vi "打码软件.vi"() -> ()   [LabVIEW 2014]
uses:
  <vilib>/Instr/_visa.llb/VISA Configure Serial Port (Instr).vi
  <vilib>/ptbypt/NI_PtbyPt.lvlib
panel:
  in  "监控":bool
  out "选项卡控件":enum32{"主选项卡", "监控"}(tab)
  in  "输入打标码后五位\n如：S0001":string
  in  "确定":bool
  out "当前打标码":string
  in  "手动打标":bool
  in  "停止":bool
  in  "退出":bool
  in  "PLC状态":bool
  out "串口通讯":bool
  out "PLC通讯":bool
  in  "返回":bool
  out "初始化回复":string
  out "打标模式回复":string
  out "初始条码":string
  out "打标V1写入回复":string
  out "打标V3写入回复":string
  out "开始打标写入回复":string
  out "停止打标回复":string
  in  "自动打标":bool
  out "错误输出 2":errorcluster caption="错误输出"
  out "元素":u32
  out "初始化文件回复":string
  out "打标V2写入回复":string
  out "枚举":T1
  # "SIC 打 标 软 件"
  # "自定义条码"
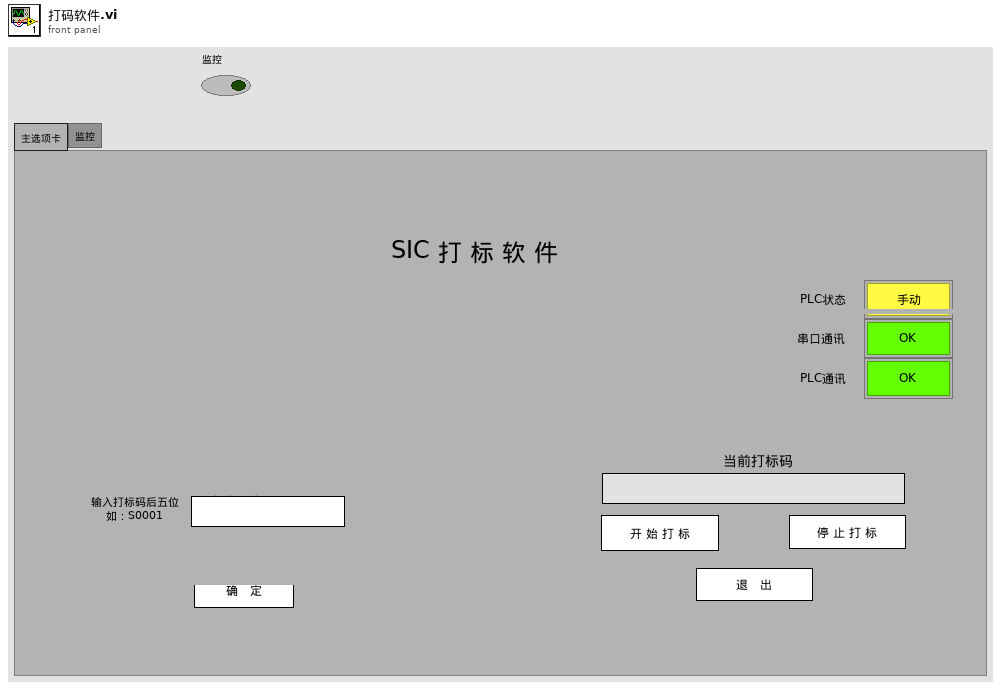
[diagram p1: front panel]
types:
  T1 = typedef "控件 1.ctl" = enum16{"通讯连接", "读PLC指令", "串口连接", "初始化", "打标模式", "事件", "错误", "退出"}
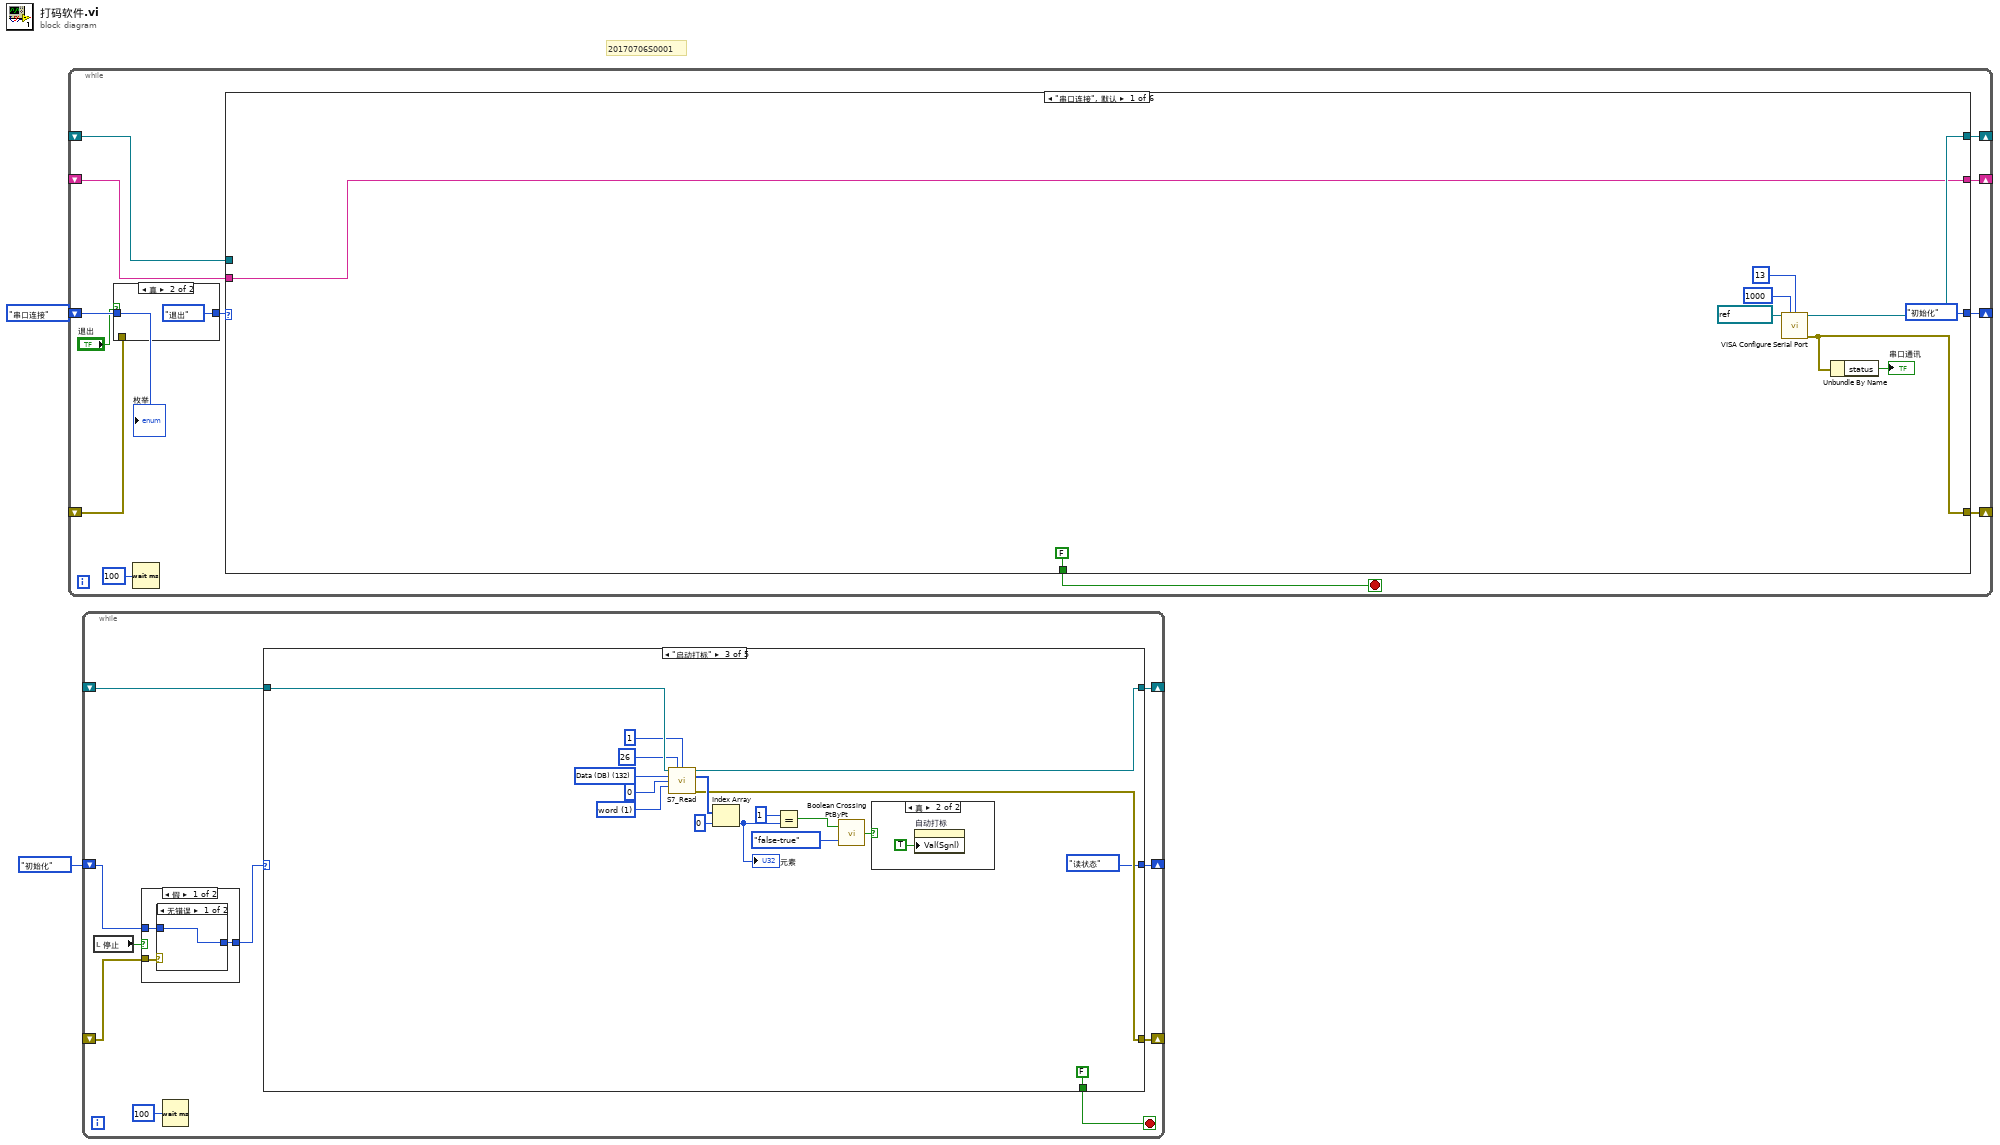
[diagram p0: block diagram]
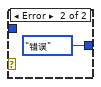
[diagram p2: hidden frame]
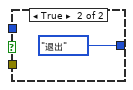
[diagram p3: hidden frame]
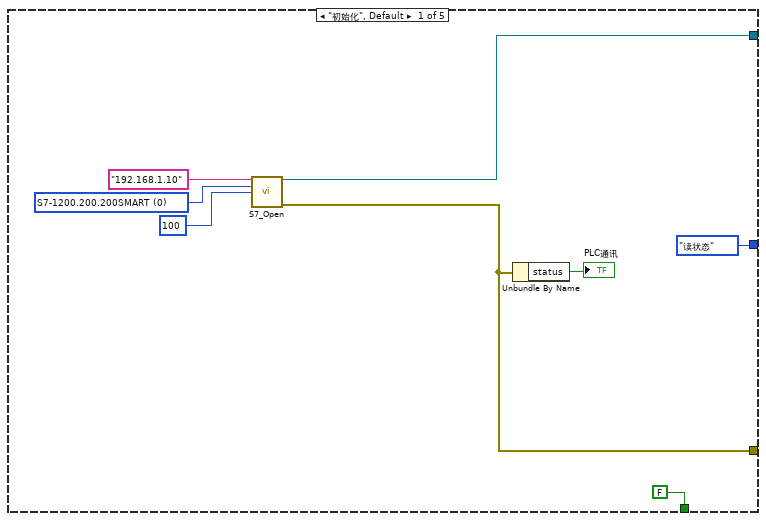
[diagram p4: hidden frame]
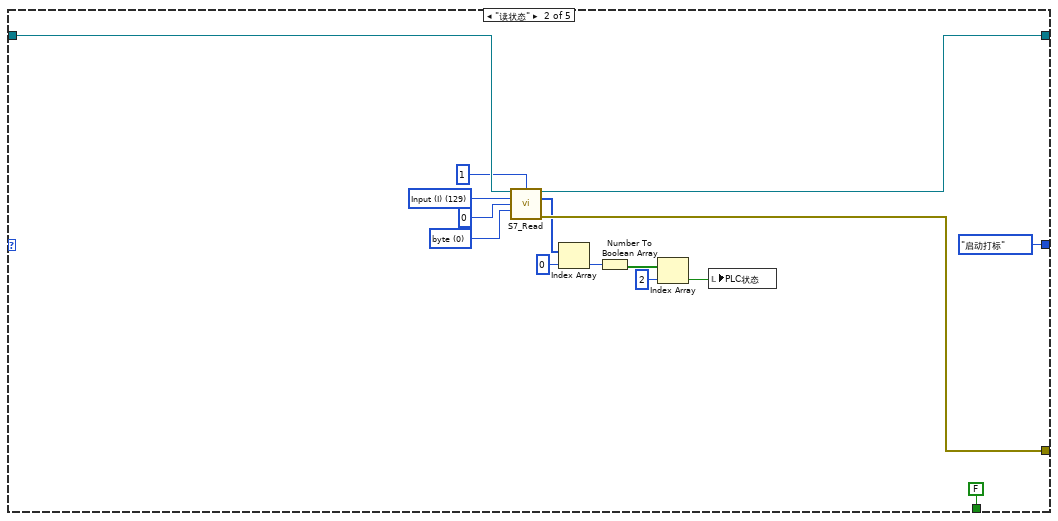
[diagram p5: hidden frame]
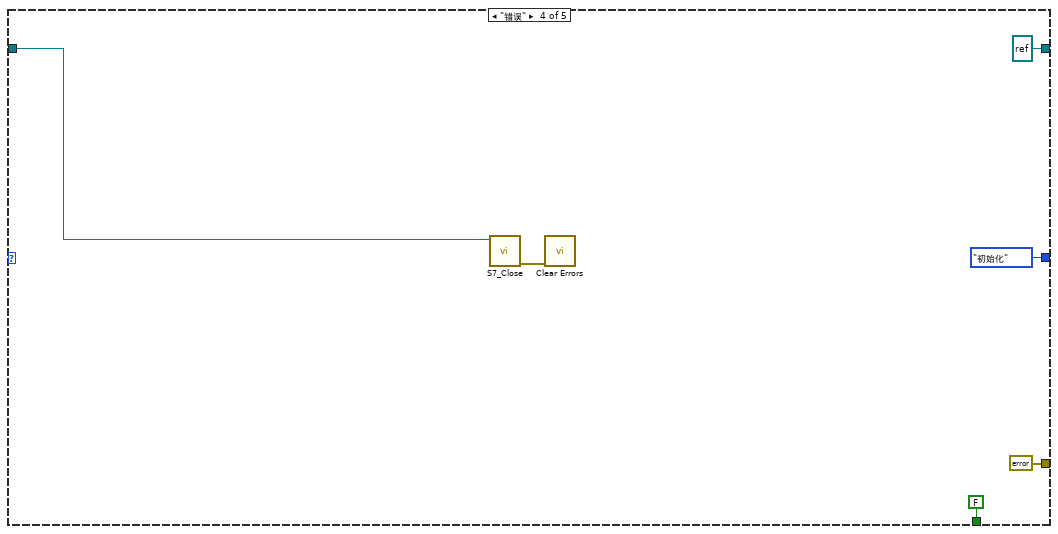
[diagram p7: hidden frame]
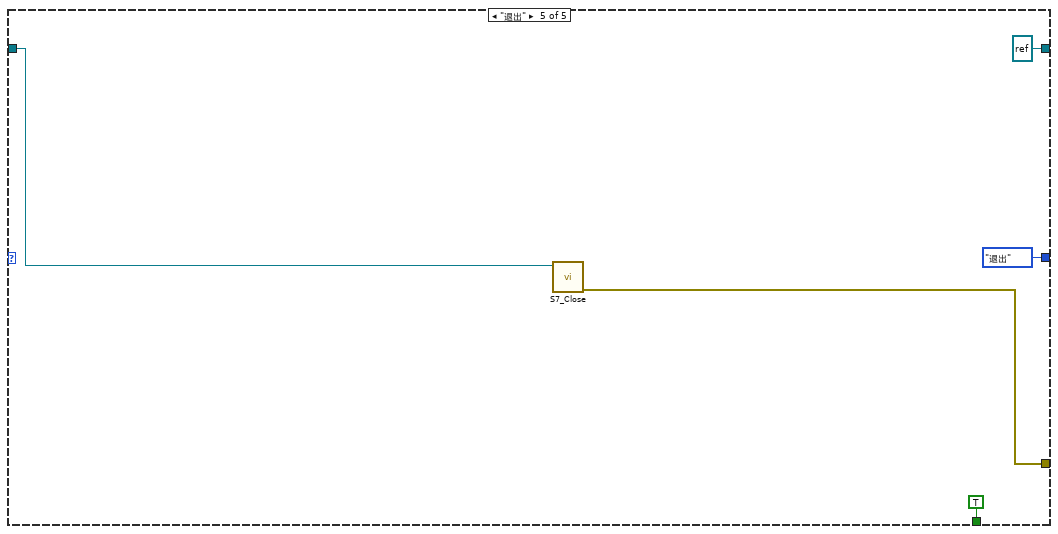
[diagram p8: hidden frame]
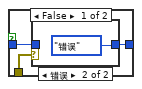
[diagram p9: hidden frame]
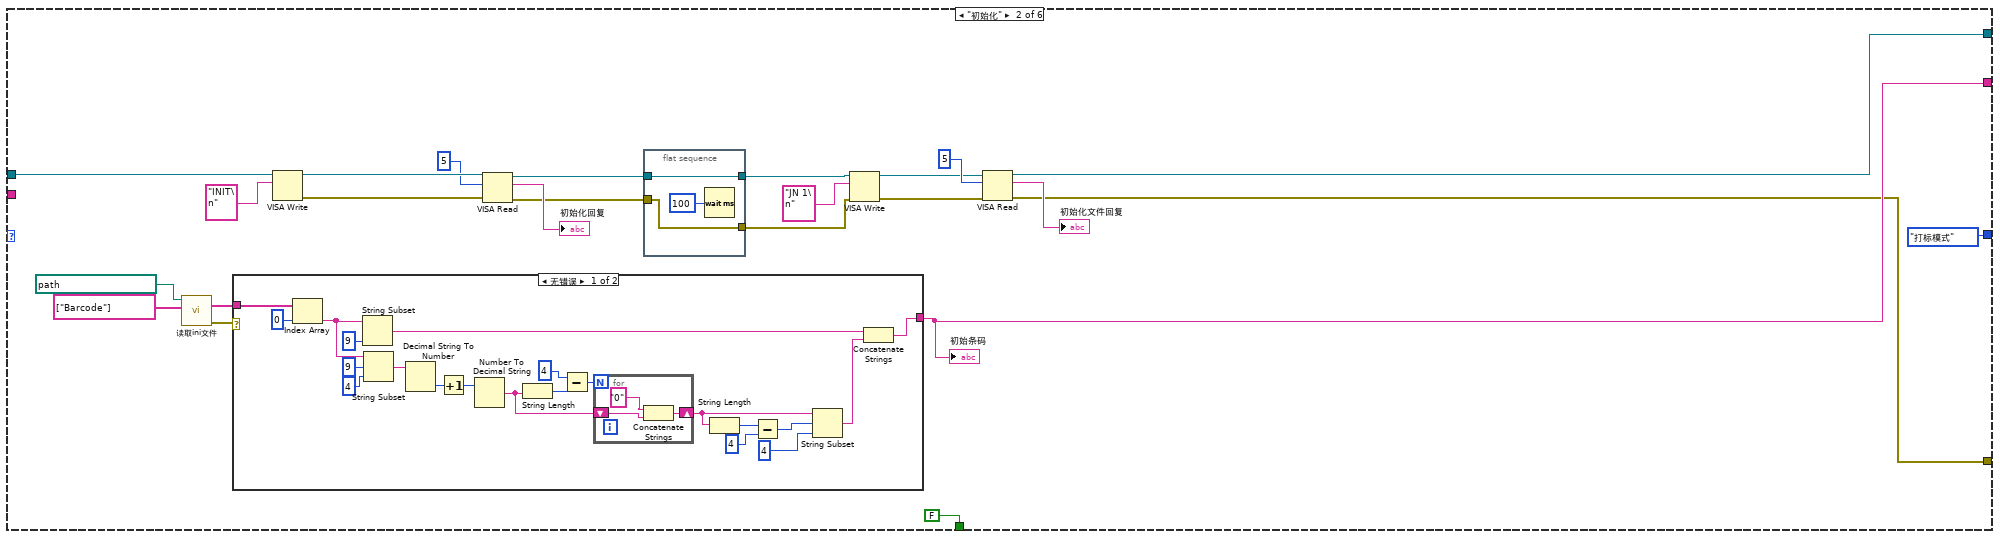
[diagram p11: hidden frame]
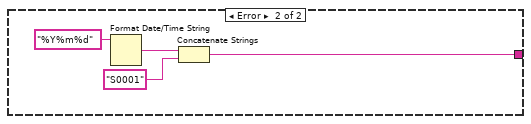
[diagram p12: hidden frame]
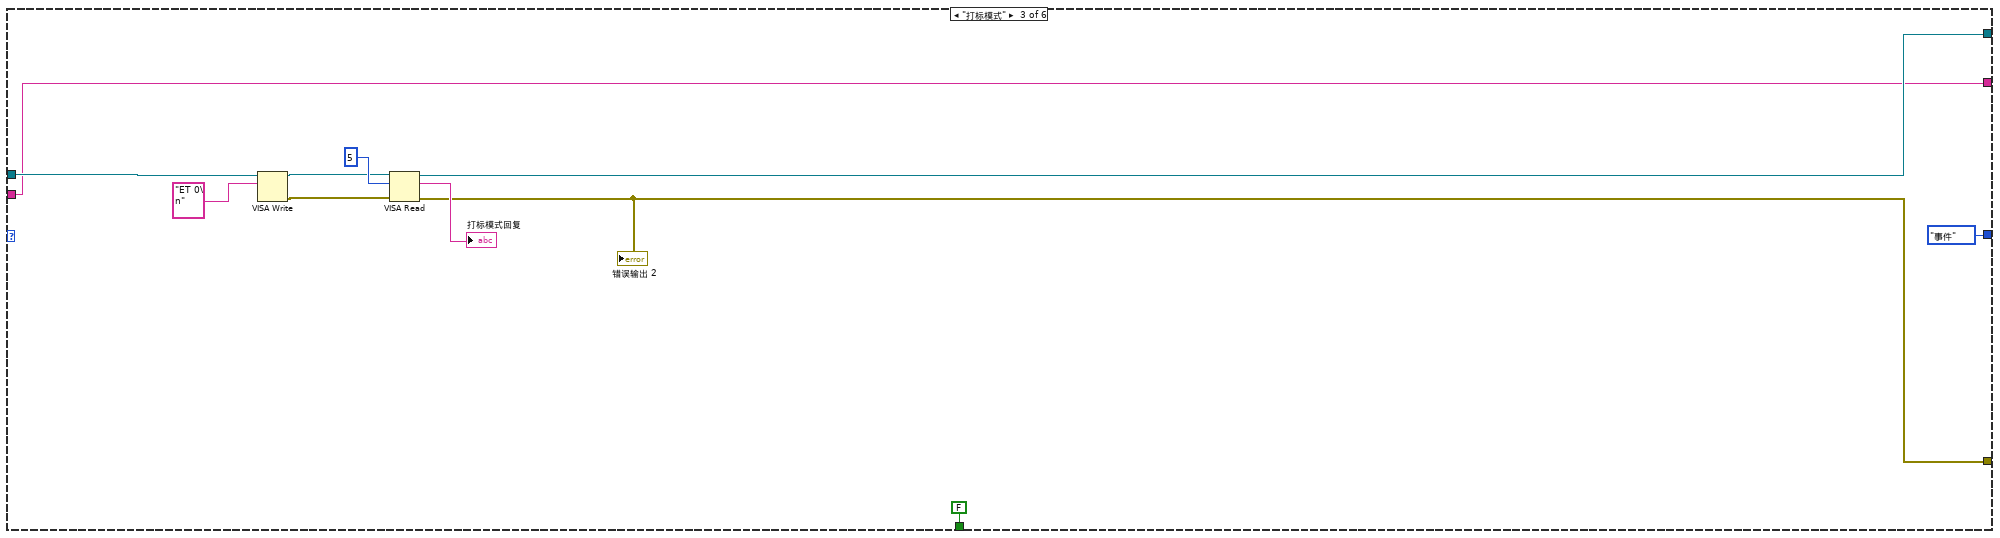
[diagram p13: hidden frame]
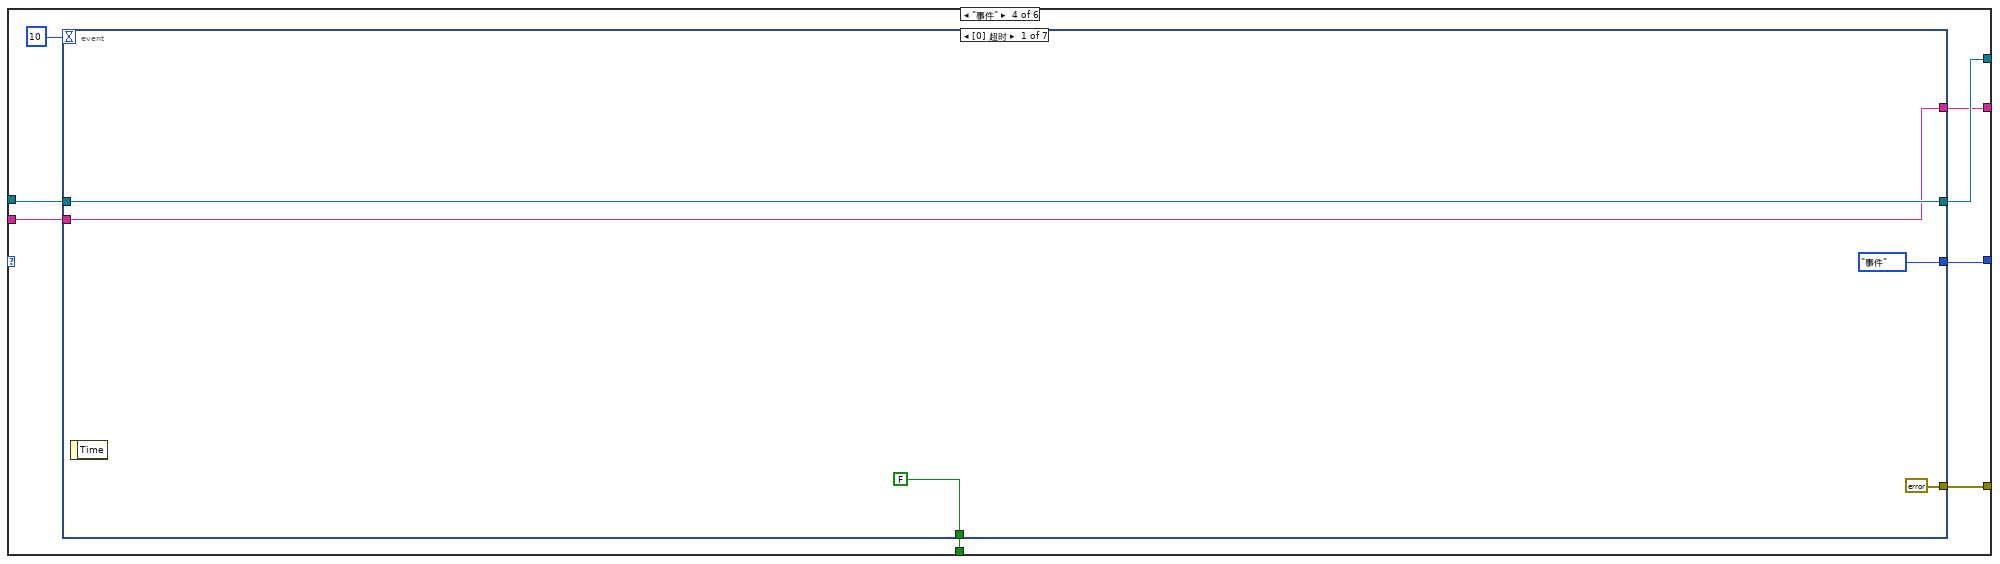
[diagram p14: hidden frame]
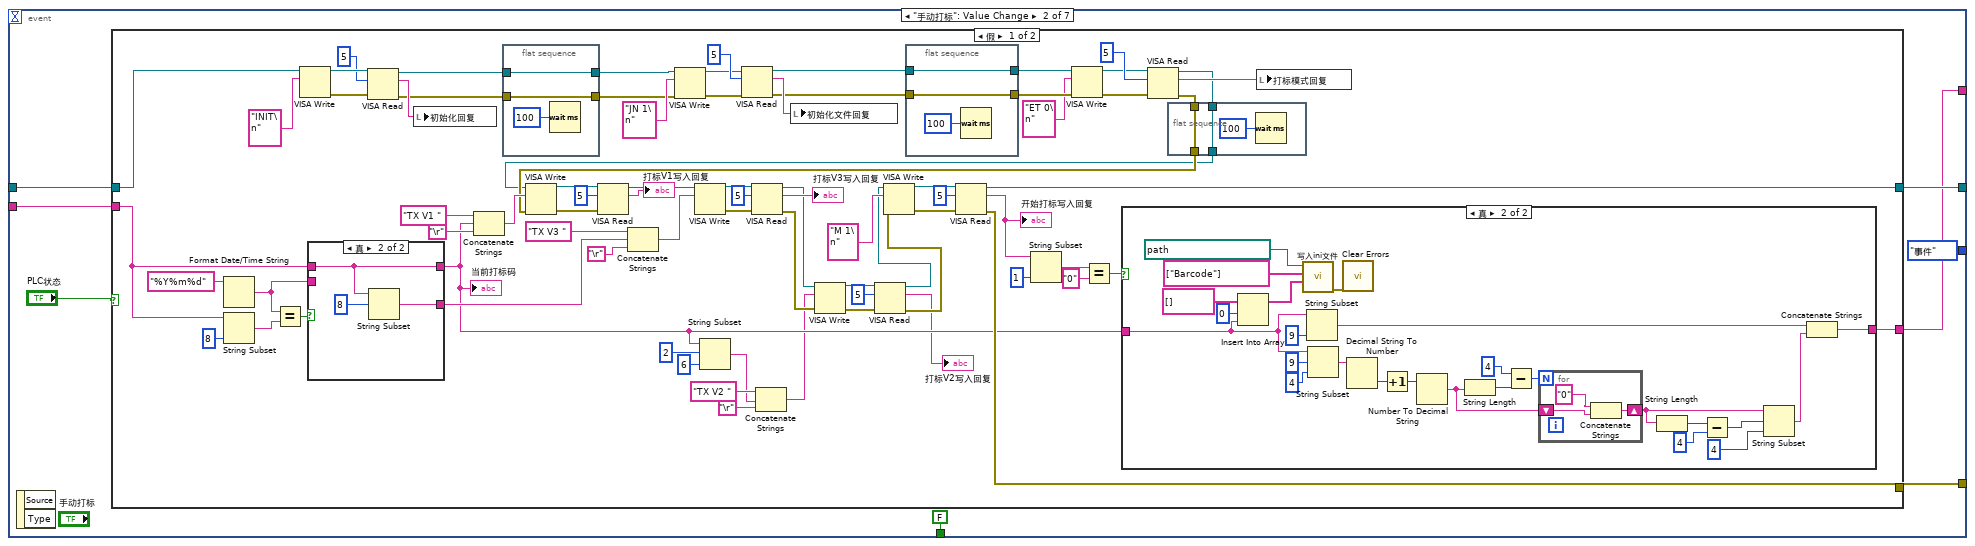
[diagram p15: hidden frame]
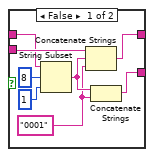
[diagram p17: hidden frame]
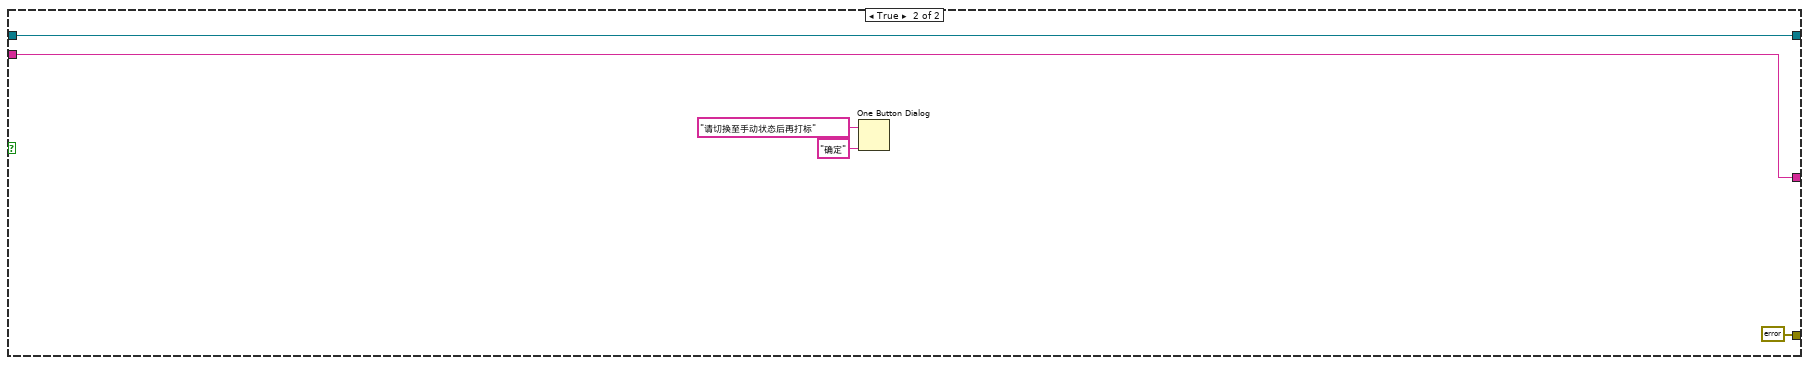
[diagram p18: hidden frame]
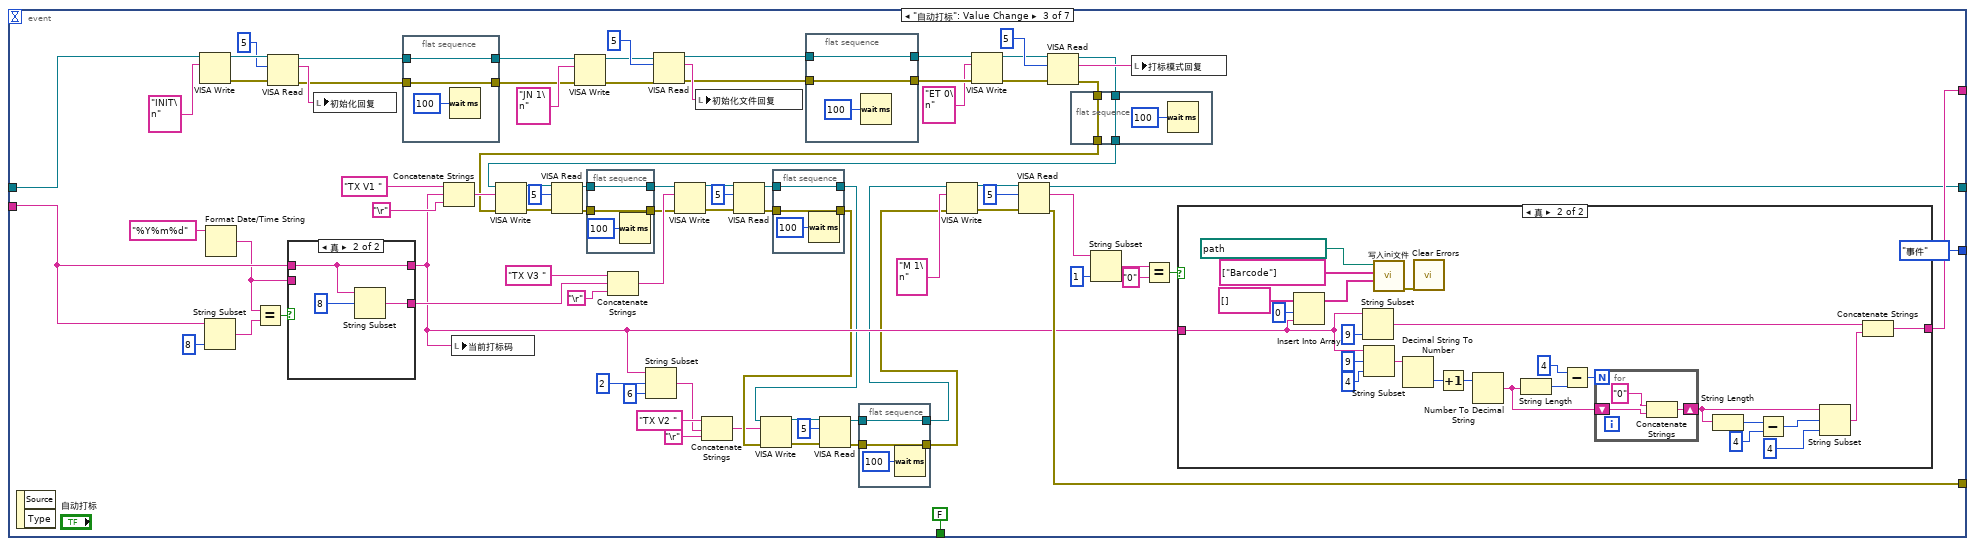
[diagram p19: hidden frame]
diagram:
  # "20170706S0001"
  n1 = while {
    shift-right: [w9] -> _
    shift-left: 控件_1."串口连接" -> [w14]
    shift-right: [w10] -> _
    shift-left: _ -> [w13]
    shift-right: [w11] -> _
    shift-left: _ -> [w8]
    shift-right: [w7] -> _
    shift-left: _ -> [w5]
    stop <- w6 stop-if-true
    n2 = case shown="真" "退出" {
      tunnel: w14 -> [w17 _]
      tunnel: w13 -> [w16 _]
      tunnel: [w15 控件_1."退出"] -> w12
      frame False {
        n3 = case shown="错误" w16 {
          tunnel: w17 -> [w18 _]
          tunnel: [w18 控件_1."错误"] -> w15
          frame No Error {
          }
          frame Error {
          }
        }
      }
      frame True {
      }
    }
    n4 = Wait (ms)(milliseconds to wait=u32 100 ("等待时间（毫秒）")) -> ()  [unwired: 1 out]
    n5 = case shown="\"串口连接\", 默认" w12 {
      tunnel: [w27 w31 w87 w99 refnum<visa-resource-name> refnum ("VISA resource name out") refnum<visa-resource-name> refnum ("VISA resource name out")] -> w11
      tunnel: [w24 w30 w88 w100 errorcluster {"status"=FALSE, "code"=0, "source"=""} ("error out") errorcluster {"status"=FALSE, "code"=0, "source"=""} ("error out")] -> w10
      tunnel: [控件_1."初始化" 控件_1."打标模式" 控件_1."事件" w97 控件_1."串口连接" 控件_1."退出"] -> w9
      tunnel: w8 -> [_ w53 w94 w102 w425 w431]
      tunnel: [w22 w42 w85 w98 w423 ""] -> w7
      tunnel: [FALSE FALSE FALSE w96 FALSE TRUE] -> w6
      tunnel: w5 -> [w22 _ w85 w101 w423 _]
      frame "串口连接", Default {
        n6 = call-poly "VISA Configure Serial Port"("VISA resource name"=refnum<visa-resource-name> "COM1", "timeout (10sec)"=u32 1000, "termination char\n(0xA = '\\n' = LF)"=u8 13 ("termination char\n(0xA = '\\n' = LF)")) -> ("VISA resource name out"=w27:refnum<visa-resource-name>, "error out"=w24:errorcluster)  [unwired: 11 in]
        n7 = Unbundle By Name(w24) -> ("status"=→"串口通讯":bool)
      }
      frame "初始化" {
        n8 = call "读取ini文件.vi"("名称"=string[] ["Barcode"], "configuration file path"=path "D:/初始化文件/10.ini") -> ("error out"=w43:errorcluster, "值"=w44:string[])  [unwired: 8 in]
        n9 = case shown="无错误" w43 {
          tunnel: w44 -> [w77 _]
          tunnel: [w57 w82] -> w42
          frame No Error {
            n10 = Index Array(array=w77, index=0 ("索引")) -> (element=w58:string)
            n11 = String Subset(string=w58, length (rest)=9 ("长度（剩余）")) -> (substring=w60:string)  [unwired: 1 in]
            n12 = String Subset(string=w58, offset (0)=9 ("偏移量(0)"), length (rest)=4 ("长度（剩余）")) -> (substring=w63:string)
            n13 = Decimal String To Number(string=w63) -> (number=w62:i32)  [unwired: 2 in, 1 out]
            n14 = Increment(x=w62) -> (x+1=w61:i32)
            n15 = Number To Decimal String(number=w61) -> (decimal integer string=w67:string)  [unwired: 1 in]
            n16 = String Length(string=w67) -> (length=w64:i32)
            n17 = Subtract(x=4, y=w64) -> (x-y=w66:i32)
            n18 = for {
              N: w66 -> [_]
              shift-right: [w80] -> w69
              shift-left: w67 -> [w79]
              n19 = Concatenate Strings("0" ("字符串"), w79) -> (w80:string)
            }
            n20 = String Length(string=w69) -> (length=w70:i32)
            n21 = Subtract(x=w70, y=4 ("x")) -> (x-y=w72:i32)
            n22 = String Subset(string=w69, offset (0)=w72, length (rest)=4 ("长度（剩余）")) -> (substring=w59:string)
            n23 = Concatenate Strings(w60, w59) -> (w57:string)
          }
          frame Error {
            n24 = Format Date/Time String(time format string (%c)="%Y%m%d" ("时间格式字符串(%c)")) -> (date/time string=w81:string)  [unwired: 2 in]
            n25 = Concatenate Strings(w81, "S0001" ("字符串")) -> (w82:string)
          }
        }
        "初始条码" <- w42
        n26 = VISA Write(VISA resource name=w53, write buffer="INIT\n" ("写入缓冲区")) -> (VISA resource name out=w50:refnum<visa-resource-name>, error out=w49:errorcluster)  [unwired: 1 in, 1 out]
        n27 = VISA Read(VISA resource name=w50, byte count=u32 5 ("字节总数"), error in (no error)=w49) -> (VISA resource name out=w37:refnum<visa-resource-name>, read buffer=→"初始化回复":string, error out=w35:errorcluster)  [unwired: 1 out]
        n28 = flat-sequence {
          tunnel: [w56] -> w36
          tunnel: w37 -> [w56]
          tunnel: w35 -> [w55]
          tunnel: [w55] -> w34
          frame #0 {
            n29 = Wait (ms)(milliseconds to wait=u32 100 ("等待时间（毫秒）")) -> ()  [unwired: 1 out]
          }
        }
        n30 = VISA Write(VISA resource name=w36, write buffer="JN 1\n" ("写入缓冲区"), error in (no error)=w34) -> (VISA resource name out=w33:refnum<visa-resource-name>, error out=w32:errorcluster)  [unwired: 1 out]
        n31 = VISA Read(VISA resource name=w33, byte count=u32 5 ("字节总数"), error in (no error)=w32) -> (VISA resource name out=w31:refnum<visa-resource-name>, read buffer=→"初始化文件回复":string, error out=w30:errorcluster)  [unwired: 1 out]
      }
      frame "打标模式" {
        n32 = VISA Write(VISA resource name=w94, write buffer="ET 0\n" ("写入缓冲区")) -> (VISA resource name out=w89:refnum<visa-resource-name>, error out=w90:errorcluster)  [unwired: 1 in, 1 out]
        n33 = VISA Read(VISA resource name=w89, byte count=u32 5 ("字节总数"), error in (no error)=w90) -> (VISA resource name out=w87:refnum<visa-resource-name>, read buffer=→"打标模式回复":string, error out=w88:errorcluster)  [unwired: 1 out]
        "错误输出 2" <- w88
      }
      frame "事件" {
        n34 = event shown="[0] 超时" {
          selector: _ -> [_ _ _ _ _ _ _]
          dyn-events: _ -> [_ _ _ _ _ _ _]
          timeout: 10 -> [_ _ _ _ _ _ _]
          tunnel: w102 -> [w108 w116 w274 w395 w404 w412 w417]
          tunnel: w101 -> [w107 w115 w302 w391 _ w413 w416]
          tunnel: [errorcluster {"status"=FALSE, "code"=0, "source"=""} ("error out") w114 w301 w392 errorcluster {"status"=FALSE, "code"=0, "source"=""} ("error out") errorcluster {"status"=FALSE, "code"=0, "source"=""} ("error out") errorcluster {"status"=FALSE, "code"=0, "source"=""} ("error out")] -> w100
          tunnel: [w108 w113 w299 w393 w404 w412 w417] -> w99
          tunnel: [w107 w112 w300 w391 w405 w413 w416] -> w98
          tunnel: [控件_1."事件" 控件_1."事件" 控件_1."事件" 控件_1."事件" 控件_1."事件" 控件_1."事件" 控件_1."事件"] -> w97
          tunnel: [FALSE FALSE FALSE FALSE FALSE FALSE FALSE] -> w96
          event Timeout {
            n35 = event-data() -> ()  [unwired: 1 in, 1 out]
          }
          event "手动打标": Value Change {
            n36 = event-data() -> ()  [unwired: 1 in, 2 out]
            n37 = case shown="假" "PLC状态" {
              tunnel: w116 -> [w136 w246]
              tunnel: w115 -> [w185 w247]
              tunnel: [w164 errorcluster {"status"=FALSE, "code"=0, "source"=""} ("error out")] -> w114
              tunnel: [w163 w246] -> w113
              tunnel: [w162 w247] -> w112
              frame False {
                n38 = Format Date/Time String(time format string (%c)="%Y%m%d" ("时间格式字符串(%c)")) -> (date/time string=w161:string)  [unwired: 2 in]
                n39 = String Subset(string=w185, length (rest)=8 ("长度（剩余）")) -> (substring=w187:string)  [unwired: 1 in]
                n40 = Equal?(x=w161, y=w187) -> (x = y?=w186:bool)
                n41 = VISA Write(VISA resource name=w136, write buffer="INIT\n" ("写入缓冲区")) -> (VISA resource name out=w147:refnum<visa-resource-name>, error out=w146:errorcluster)  [unwired: 1 in, 1 out]
                n42 = case shown="真" w186 {
                  tunnel: w185 -> [w238 w242]
                  tunnel: [w235 w242] -> w124
                  tunnel: [w234 w240] -> w160
                  tunnel: w161 -> [w239 _]
                  frame False {
                    w232 = "0001"
                    n43 = String Subset(string=w238, offset (0)=8 ("偏移量(0)"), length (rest)=1 ("长度（剩余）")) -> (substring=w233:string)
                    n44 = Concatenate Strings(w239, w233, w232) -> (w235:string)
                    n45 = Concatenate Strings(w233, w232) -> (w234:string)
                  }
                  frame True {
                    n46 = String Subset(string=w242, offset (0)=8 ("偏移量(0)")) -> (substring=w240:string)  [unwired: 1 in]
                  }
                }
                "当前打标码" <- w124
                n47 = VISA Read(VISA resource name=w147, byte count=u32 5 ("字节总数"), error in (no error)=w146) -> (VISA resource name out=w142:refnum<visa-resource-name>, read buffer=w157:string, error out=w140:errorcluster)  [unwired: 1 out]
                n48 = local write "初始化回复"(w157) -> ()
                n49 = Concatenate Strings("TX V1 " ("写入缓冲区"), w124, "\r") -> (w182:string)
                n50 = flat-sequence {
                  tunnel: [w202] -> w141
                  tunnel: w142 -> [w202]
                  tunnel: w140 -> [w201]
                  tunnel: [w201] -> w139
                  frame #0 {
                    n51 = Wait (ms)(milliseconds to wait=u32 100 ("等待时间（毫秒）")) -> ()  [unwired: 1 out]
                  }
                }
                n52 = VISA Write(VISA resource name=w132, write buffer=w182, error in (no error)=w134) -> (VISA resource name out=w193:refnum<visa-resource-name>, error out=w192:errorcluster)  [unwired: 1 out]
                n53 = VISA Read(VISA resource name=w193, byte count=u32 5 ("字节总数"), error in (no error)=w192) -> (VISA resource name out=w175:refnum<visa-resource-name>, read buffer=→"打标V1写入回复":string)  [unwired: 2 out]
                n54 = Concatenate Strings("TX V3 " ("写入缓冲区"), w160, "\r") -> (w181:string)
                n55 = VISA Write(VISA resource name=w141, write buffer="JN 1\n" ("写入缓冲区"), error in (no error)=w139) -> (VISA resource name out=w138:refnum<visa-resource-name>, error out=w137:errorcluster)  [unwired: 1 out]
                n56 = VISA Write(VISA resource name=w175, write buffer=w181) -> (VISA resource name out=w176:refnum<visa-resource-name>, error out=w177:errorcluster)  [unwired: 1 in, 1 out]
                n57 = String Subset(string=w124, offset (0)=2 ("偏移量(0)"), length (rest)=6 ("长度（剩余）")) -> (substring=w120:string)
                n58 = VISA Read(VISA resource name=w138, byte count=u32 5 ("字节总数"), error in (no error)=w137) -> (VISA resource name out=w153:refnum<visa-resource-name>, read buffer=w158:string, error out=w155:errorcluster)  [unwired: 1 out]
                n59 = VISA Read(VISA resource name=w176, byte count=u32 5 ("字节总数"), error in (no error)=w177) -> (VISA resource name out=w127:refnum<visa-resource-name>, read buffer=→"打标V3写入回复":string, error out=w128:errorcluster)  [unwired: 1 out]
                n60 = Concatenate Strings("TX V2 " ("写入缓冲区"), w120, "\r") -> (w119:string)
                n61 = local write "初始化文件回复"(w158) -> ()
                n62 = VISA Write(VISA resource name=w127, write buffer=w119, error in (no error)=w128) -> (VISA resource name out=w131:refnum<visa-resource-name>, error out=w130:errorcluster)  [unwired: 1 out]
                n63 = VISA Read(VISA resource name=w131, byte count=u32 5 ("字节总数"), error in (no error)=w130) -> (VISA resource name out=w126:refnum<visa-resource-name>, read buffer=→"打标V2写入回复":string, error out=w125:errorcluster)  [unwired: 1 out]
                n64 = VISA Write(VISA resource name=w126, write buffer="M 1\n" ("写入缓冲区"), error in (no error)=w125) -> (VISA resource name out=w173:refnum<visa-resource-name>, error out=w172:errorcluster)  [unwired: 1 out]
                n65 = flat-sequence {
                  tunnel: [w199] -> w154
                  tunnel: w153 -> [w199]
                  tunnel: [w198] -> w156
                  tunnel: w155 -> [w198]
                  frame #0 {
                    n66 = Wait (ms)(milliseconds to wait=u32 100 ("等待时间（毫秒）")) -> ()  [unwired: 1 out]
                  }
                }
                n67 = VISA Read(VISA resource name=w173, byte count=u32 5 ("字节总数"), error in (no error)=w172) -> (VISA resource name out=w163:refnum<visa-resource-name>, read buffer=w169:string, error out=w164:errorcluster)  [unwired: 1 out]
                "开始打标写入回复" <- w169
                n68 = String Subset(string=w169, length (rest)=1 ("长度（剩余）")) -> (substring=w167:string)  [unwired: 1 in]
                n69 = VISA Write(VISA resource name=w154, write buffer="ET 0\n" ("写入缓冲区"), error in (no error)=w156) -> (VISA resource name out=w149:refnum<visa-resource-name>, error out=w150:errorcluster)  [unwired: 1 out]
                n70 = Equal?(x=w167, y="0") -> (x = y?=w165:bool)
                n71 = case shown="真" w165 {
                  tunnel: w124 -> [w203 w205]
                  tunnel: [w203 w204] -> w162
                  frame False {
                  }
                  frame True {
                    n72 = Insert Into Array(array=string[] [] ("数组"), index=0 ("索引"), new element=w205) -> (w225:string[])
                    n73 = call "写入ini文件.vi"("值"=w225, "名称"=string[] ["Barcode"], "configuration file path"=path "D:/初始化文件/10.ini") -> ("error out"=w228:errorcluster)  [unwired: 8 in]
                    n74 = String Subset(string=w205, length (rest)=9 ("长度（剩余）")) -> (substring=w207:string)  [unwired: 1 in]
                    n75 = String Subset(string=w205, offset (0)=9 ("偏移量(0)"), length (rest)=4 ("长度（剩余）")) -> (substring=w210:string)
                    n76 = call <vilib>:"Clear Errors.vi"("error in (no error)"=w228) -> ()  [unwired: 5 in, 2 out]
                    n77 = Decimal String To Number(string=w210) -> (number=w209:i32)  [unwired: 2 in, 1 out]
                    n78 = Increment(x=w209) -> (x+1=w208:i32)
                    n79 = Number To Decimal String(number=w208) -> (decimal integer string=w214:string)  [unwired: 1 in]
                    n80 = String Length(string=w214) -> (length=w211:i32)
                    n81 = Subtract(x=4, y=w211) -> (x-y=w213:i32)
                    n82 = for {
                      N: w213 -> [_]
                      shift-right: [w231] -> w216
                      shift-left: w214 -> [w230]
                      n83 = Concatenate Strings("0" ("字符串"), w230) -> (w231:string)
                    }
                    n84 = String Length(string=w216) -> (length=w217:i32)
                    n85 = Subtract(x=w217, y=4 ("x")) -> (x-y=w219:i32)
                    n86 = String Subset(string=w216, offset (0)=w219, length (rest)=4 ("长度（剩余）")) -> (substring=w206:string)
                    n87 = Concatenate Strings(w207, w206) -> (w204:string)
                  }
                }
                n88 = VISA Read(VISA resource name=w149, byte count=u32 5 ("字节总数"), error in (no error)=w150) -> (VISA resource name out=w133:refnum<visa-resource-name>, read buffer=w159:string, error out=w135:errorcluster)  [unwired: 1 out]
                n89 = flat-sequence {
                  tunnel: w133 -> [w196]
                  tunnel: [w196] -> w132
                  tunnel: w135 -> [w195]
                  tunnel: [w195] -> w134
                  frame #0 {
                    n90 = Wait (ms)(milliseconds to wait=u32 100 ("等待时间（毫秒）")) -> ()  [unwired: 1 out]
                  }
                }
                n91 = local write "打标模式回复"(w159) -> ()
              }
              frame True {
                n92 = One Button Dialog(message="请切换至手动状态后再打标" ("消息"), button name ("OK")="确定" ("按钮名称（“确定”）")) -> ()  [unwired: 1 out]
              }
            }
          }
          event "自动打标": Value Change {
            n93 = event-data() -> ()  [unwired: 1 in, 2 out]
            n94 = VISA Write(VISA resource name=w274, write buffer="INIT\n" ("写入缓冲区")) -> (VISA resource name out=w285:refnum<visa-resource-name>, error out=w284:errorcluster)  [unwired: 1 in, 1 out]
            n95 = String Subset(string=w302, length (rest)=8 ("长度（剩余）")) -> (substring=w323:string)  [unwired: 1 in]
            n96 = Format Date/Time String(time format string (%c)="%Y%m%d" ("时间格式字符串(%c)")) -> (date/time string=w298:string)  [unwired: 2 in]
            n97 = Equal?(x=w298, y=w323) -> (x = y?=w322:bool)
            n98 = VISA Read(VISA resource name=w285, byte count=u32 5 ("字节总数"), error in (no error)=w284) -> (VISA resource name out=w280:refnum<visa-resource-name>, read buffer=w295:string, error out=w278:errorcluster)  [unwired: 1 out]
            n99 = case shown="真" w322 {
              tunnel: w302 -> [w384 w388]
              tunnel: [w381 w388] -> w260
              tunnel: [w380 w386] -> w312
              tunnel: w298 -> [w385 _]
              frame False {
                w378 = "0001"
                n100 = String Subset(string=w384, offset (0)=8 ("偏移量(0)"), length (rest)=1 ("长度（剩余）")) -> (substring=w379:string)
                n101 = Concatenate Strings(w385, w379, w378) -> (w381:string)
                n102 = Concatenate Strings(w379, w378) -> (w380:string)
              }
              frame True {
                n103 = String Subset(string=w388, offset (0)=8 ("偏移量(0)")) -> (substring=w386:string)  [unwired: 1 in]
              }
            }
            n104 = local write "初始化回复"(w295) -> ()
            n105 = flat-sequence {
              tunnel: [w348] -> w279
              tunnel: w280 -> [w348]
              tunnel: w278 -> [w347]
              tunnel: [w347] -> w277
              frame #0 {
                n106 = Wait (ms)(milliseconds to wait=u32 100 ("等待时间（毫秒）")) -> ()  [unwired: 1 out]
              }
            }
            n107 = Concatenate Strings("TX V1 " ("写入缓冲区"), w260, "\r") -> (w319:string)
            n108 = local write "当前打标码"(w260) -> ()
            n109 = VISA Write(VISA resource name=w272, write buffer=w319, error in (no error)=w270) -> (VISA resource name out=w328:refnum<visa-resource-name>, error out=w327:errorcluster)  [unwired: 1 out]
            n110 = VISA Read(VISA resource name=w328, byte count=u32 5 ("字节总数"), error in (no error)=w327) -> (VISA resource name out=w269:refnum<visa-resource-name>, error out=w267:errorcluster)  [unwired: 2 out]
            n111 = VISA Write(VISA resource name=w279, write buffer="JN 1\n" ("写入缓冲区"), error in (no error)=w277) -> (VISA resource name out=w276:refnum<visa-resource-name>, error out=w275:errorcluster)  [unwired: 1 out]
            n112 = flat-sequence {
              tunnel: w269 -> [w339]
              tunnel: [w339] -> w268
              tunnel: w267 -> [w338]
              tunnel: [w338] -> w266
              frame #0 {
                n113 = Wait (ms)(milliseconds to wait=u32 100 ("等待时间（毫秒）")) -> ()  [unwired: 1 out]
              }
            }
            n114 = Concatenate Strings("TX V3 " ("写入缓冲区"), w312, "\r") -> (w318:string)
            n115 = String Subset(string=w260, offset (0)=2 ("偏移量(0)"), length (rest)=6 ("长度（剩余）")) -> (substring=w261:string)
            n116 = VISA Read(VISA resource name=w276, byte count=u32 5 ("字节总数"), error in (no error)=w275) -> (VISA resource name out=w291:refnum<visa-resource-name>, read buffer=w296:string, error out=w293:errorcluster)  [unwired: 1 out]
            n117 = VISA Write(VISA resource name=w268, write buffer=w318, error in (no error)=w266) -> (VISA resource name out=w313:refnum<visa-resource-name>, error out=w314:errorcluster)  [unwired: 1 out]
            n118 = local write "初始化文件回复"(w296) -> ()
            n119 = Concatenate Strings("TX V2 " ("写入缓冲区"), w261, "\r") -> (w252:string)
            n120 = VISA Read(VISA resource name=w313, byte count=u32 5 ("字节总数"), error in (no error)=w314) -> (VISA resource name out=w264:refnum<visa-resource-name>, error out=w265:errorcluster)  [unwired: 2 out]
            n121 = VISA Write(VISA resource name=w254, write buffer=w252, error in (no error)=w253) -> (VISA resource name out=w257:refnum<visa-resource-name>, error out=w256:errorcluster)  [unwired: 1 out]
            n122 = flat-sequence {
              tunnel: w264 -> [w336]
              tunnel: [w336] -> w254
              tunnel: w265 -> [w335]
              tunnel: [w335] -> w253
              frame #0 {
                n123 = Wait (ms)(milliseconds to wait=u32 100 ("等待时间（毫秒）")) -> ()  [unwired: 1 out]
              }
            }
            n124 = flat-sequence {
              tunnel: [w345] -> w292
              tunnel: w291 -> [w345]
              tunnel: [w344] -> w294
              tunnel: w293 -> [w344]
              frame #0 {
                n125 = Wait (ms)(milliseconds to wait=u32 100 ("等待时间（毫秒）")) -> ()  [unwired: 1 out]
              }
            }
            n126 = VISA Read(VISA resource name=w257, byte count=u32 5 ("字节总数"), error in (no error)=w256) -> (VISA resource name out=w259:refnum<visa-resource-name>, error out=w258:errorcluster)  [unwired: 2 out]
            n127 = flat-sequence {
              tunnel: w259 -> [w333]
              tunnel: [w333] -> w251
              tunnel: w258 -> [w332]
              tunnel: [w332] -> w250
              frame #0 {
                n128 = Wait (ms)(milliseconds to wait=u32 100 ("等待时间（毫秒）")) -> ()  [unwired: 1 out]
              }
            }
            n129 = VISA Write(VISA resource name=w251, write buffer="M 1\n" ("写入缓冲区"), error in (no error)=w250) -> (VISA resource name out=w311:refnum<visa-resource-name>, error out=w310:errorcluster)  [unwired: 1 out]
            n130 = VISA Write(VISA resource name=w292, write buffer="ET 0\n" ("写入缓冲区"), error in (no error)=w294) -> (VISA resource name out=w287:refnum<visa-resource-name>, error out=w288:errorcluster)  [unwired: 1 out]
            n131 = VISA Read(VISA resource name=w311, byte count=u32 5 ("字节总数"), error in (no error)=w310) -> (VISA resource name out=w299:refnum<visa-resource-name>, read buffer=w307:string, error out=w301:errorcluster)  [unwired: 1 out]
            n132 = VISA Read(VISA resource name=w287, byte count=u32 5 ("字节总数"), error in (no error)=w288) -> (VISA resource name out=w273:refnum<visa-resource-name>, read buffer=w297:string, error out=w271:errorcluster)  [unwired: 1 out]
            n133 = flat-sequence {
              tunnel: w273 -> [w342]
              tunnel: [w342] -> w272
              tunnel: w271 -> [w341]
              tunnel: [w341] -> w270
              frame #0 {
                n134 = Wait (ms)(milliseconds to wait=u32 100 ("等待时间（毫秒）")) -> ()  [unwired: 1 out]
              }
            }
            n135 = String Subset(string=w307, length (rest)=1 ("长度（剩余）")) -> (substring=w305:string)  [unwired: 1 in]
            n136 = local write "打标模式回复"(w297) -> ()
            n137 = Equal?(x=w305, y="0") -> (x = y?=w303:bool)
            n138 = case shown="真" w303 {
              tunnel: w260 -> [w349 w351]
              tunnel: [w349 w350] -> w300
              frame False {
              }
              frame True {
                n139 = Insert Into Array(array=string[] [] ("数组"), index=0 ("索引"), new element=w351) -> (w371:string[])
                n140 = String Subset(string=w351, length (rest)=9 ("长度（剩余）")) -> (substring=w353:string)  [unwired: 1 in]
                n141 = String Subset(string=w351, offset (0)=9 ("偏移量(0)"), length (rest)=4 ("长度（剩余）")) -> (substring=w356:string)
                n142 = call "写入ini文件.vi"("值"=w371, "名称"=string[] ["Barcode"], "configuration file path"=path "D:/初始化文件/10.ini") -> ("error out"=w374:errorcluster)  [unwired: 8 in]
                n143 = Decimal String To Number(string=w356) -> (number=w355:i32)  [unwired: 2 in, 1 out]
                n144 = call <vilib>:"Clear Errors.vi"("error in (no error)"=w374) -> ()  [unwired: 5 in, 2 out]
                n145 = Increment(x=w355) -> (x+1=w354:i32)
                n146 = Number To Decimal String(number=w354) -> (decimal integer string=w360:string)  [unwired: 1 in]
                n147 = String Length(string=w360) -> (length=w357:i32)
                n148 = Subtract(x=4, y=w357) -> (x-y=w359:i32)
                n149 = for {
                  N: w359 -> [_]
                  shift-right: [w377] -> w362
                  shift-left: w360 -> [w376]
                  n150 = Concatenate Strings("0" ("字符串"), w376) -> (w377:string)
                }
                n151 = String Length(string=w362) -> (length=w363:i32)
                n152 = Subtract(x=w363, y=4 ("x")) -> (x-y=w365:i32)
                n153 = String Subset(string=w362, offset (0)=w365, length (rest)=4 ("长度（剩余）")) -> (substring=w352:string)
                n154 = Concatenate Strings(w353, w352) -> (w350:string)
              }
            }
          }
          event "停止": Value Change {
            n155 = event-data() -> ()  [unwired: 1 in, 2 out]
            n156 = VISA Write(VISA resource name=w395, write buffer="M 0\n" ("写入缓冲区")) -> (VISA resource name out=w399:refnum<visa-resource-name>, error out=w398:errorcluster)  [unwired: 1 in, 1 out]
            n157 = VISA Read(VISA resource name=w399, byte count=u32 5 ("字节总数"), error in (no error)=w398) -> (VISA resource name out=w393:refnum<visa-resource-name>, read buffer=→"停止打标回复":string, error out=w392:errorcluster)  [unwired: 1 out]
          }
          event "确定": Value Change {
            n158 = event-data() -> ()  [unwired: 1 in, 2 out]
            n159 = Format Date/Time String(time format string (%c)="%Y%m%d" ("时间格式字符串(%c)")) -> (date/time string=w400:string)  [unwired: 2 in]
            n160 = Concatenate Strings(w400, "输入打标码后五位\n如：S0001") -> (w405:string)
          }
          event "监控": Value Change {
            n161 = event-data() -> ()  [unwired: 1 in, 4 out]
            "选项卡控件" <- enum32{"主选项卡", "监控"}."监控" ("选项卡控件")
          }
          event "返回": Value Change {
            n162 = event-data() -> ()  [unwired: 1 in, 4 out]
            n163 = local write "选项卡控件"(enum32{"主选项卡", "监控"}."主选项卡" ("选项卡控件")) -> ()
          }
        }
      }
      frame "错误" {
        n164 = VISA Close(VISA resource name=w425) -> ()  [unwired: 1 in, 1 out]
      }
      frame "退出" {
        n165 = VISA Close(VISA resource name=w431) -> (error out=w432:errorcluster)  [unwired: 1 in]
        n166 = call <vilib>:"Clear Errors.vi"("error in (no error)"=w432) -> ()  [unwired: 5 in, 2 out]
        n167 = control-ref of="本VI"() -> (w433:refnum<vi>)
        n168 = invoke class="VI" method="FP.Close"(reference=w433) -> ()  [unwired: 2 in, 3 out]
      }
    }
    "枚举" <- w14
  }
  n169 = while {
    shift-right: [w442] -> _
    shift-left: _ -> [w439]
    shift-right: [w441] -> _
    shift-left: _ -> [w437]
    shift-right: [w440] -> _
    shift-left: enum16{"初始化", "读状态", "启动打标", "错误", "退出"}."初始化" -> [w436]
    stop <- w438 stop-if-true
    n170 = local read "停止"() -> (w443:bool)
    n171 = case shown="假" w443 {
      tunnel: [w445 enum16{"初始化", "读状态", "启动打标", "错误", "退出"}."退出"] -> w435
      tunnel: w437 -> [w446 _]
      tunnel: w436 -> [w444 _]
      frame False {
        n172 = case shown="无错误" w446 {
          tunnel: [w447 enum16{"初始化", "读状态", "启动打标", "错误", "退出"}."错误"] -> w445
          tunnel: w444 -> [w447 _]
          frame No Error {
          }
          frame Error {
          }
        }
      }
      frame True {
      }
    }
    n173 = Wait (ms)(milliseconds to wait=u32 100 ("等待时间（毫秒）")) -> ()  [unwired: 1 out]
    n174 = case shown="\"启动打标\"" w435 {
      tunnel: [w453 w467 w483 refnum<k5> refnum ("TCP") refnum<k5> refnum ("TCP")] -> w442
      tunnel: [w452 w468 w482 errorcluster {"status"=FALSE, "code"=0, "source"=""} ("error out") w500] -> w441
      tunnel: [enum16{"初始化", "读状态", "启动打标", "错误", "退出"}."读状态" enum16{"初始化", "读状态", "启动打标", "错误", "退出"}."启动打标" enum16{"初始化", "读状态", "启动打标", "错误", "退出"}."读状态" enum16{"初始化", "读状态", "启动打标", "错误", "退出"}."初始化" enum16{"初始化", "读状态", "启动打标", "错误", "退出"}."退出"] -> w440
      tunnel: w439 -> [_ w472 w484 w496 w501]
      tunnel: [FALSE FALSE FALSE FALSE TRUE] -> w438
      frame "初始化", Default {
        w456 = u8 0 items=["S7-1200.200.200SMART"=0, "S7-300"=2, "S7-400"=3] ("PLC 系列")
        n175 = call "S7_Open.vi"("IP 地址"="192.168.1.10", "PLC 系列"=w456, "超时（MS）"=100) -> ("TCP"=w453:refnum<k5>, "error out"=w452:errorcluster)  [unwired: 10 in, 1 out]
        n176 = Unbundle By Name(w452) -> ("status"=→"PLC通讯":bool)
      }
      frame "读状态" {
        w469 = u16 0 items=["byte", "word", "Dword"] ("数据类型")
        w471 = u8 129 items=["I/O (P)"=128, "Input (I)"=129, "Output (Q)"=130, "Bit Memory (M)"=131, "Data (DB)"=132, "Instance Data (DI)"=133, "Local Data (L)"=134, "Predecessor Local Data (VL)"=135] ("寄存器类型")
        n177 = call "S7_Read.vi"("TCP"=w472, "读取长度"=u16 1, "寄存器类型"=w471, "起始地址"=u32 0, "数据类型"=w469) -> ("TCP"=w467:refnum<k5>, "数据"=w466:u32[], "error out"=w468:errorcluster)  [unwired: 7 in, 1 out]
        n178 = Index Array(array=w466, index=0 ("索引")) -> (element=w461:u32)
        n179 = Number To Boolean Array(number=w461) -> (Boolean array=w460:bool[])
        n180 = Index Array(array=w460, index=2 ("索引")) -> (element=w458:bool)
        n181 = local write "PLC状态"(w458) -> ()
      }
      frame "启动打标" {
        w487 = u16 1 items=["byte", "word", "Dword"] ("数据类型")
        w489 = u8 132 items=["I/O (P)"=128, "Input (I)"=129, "Output (Q)"=130, "Bit Memory (M)"=131, "Data (DB)"=132, "Instance Data (DI)"=133, "Local Data (L)"=134, "Predecessor Local Data (VL)"=135] ("寄存器类型")
        n182 = call "S7_Read.vi"("TCP"=w484, "DB #"=u16 26, "读取长度"=u16 1, "寄存器类型"=w489, "起始地址"=u32 0, "数据类型"=w487) -> ("TCP"=w483:refnum<k5>, "数据"=w486:u32[], "error out"=w482:errorcluster)  [unwired: 6 in, 1 out]
        n183 = Index Array(array=w486, index=0 ("索引")) -> (element=w475:u32)
        "元素" <- w475
        n184 = Equal?(x=u32 1, y=w475) -> (x = y?=w473:bool)
        n185 = call <vilib>:"Boolean Crossing PtByPt.vi"("direction"=enum16{"either", "false-true", "true-false"}."false-true", "input"=w473) -> ("crossing"=w478:bool)  [unwired: 1 in]
        n186 = case shown="真" w478 {
          frame False {
          }
          frame True {
            n187 = property on="自动打标" class="Bool (严格)"("Val(Sgnl)"=TRUE ("值(信号)")) -> ()  [unwired: 2 in, 2 out]
          }
        }
      }
      frame "错误" {
        n188 = call "S7_Close.vi"("TCP Connection Ref"=w496) -> ("error out"=w492:errorcluster)  [unwired: 10 in]
        n189 = call <vilib>:"Clear Errors.vi"("error in (no error)"=w492) -> ()  [unwired: 5 in, 2 out]
      }
      frame "退出" {
        n190 = call "S7_Close.vi"("TCP Connection Ref"=w501) -> ("error out"=w500:errorcluster)  [unwired: 10 in]
      }
    }
  }
